vi "Calibrare.vi"() -> ()   [LabVIEW 2018]
panel:
  out "Timer":dbl
  out "Timer pornire":dbl
  out "Timer finalizare calibrare":dbl
  in  "Bluetooth":refnum<visa-resource-name>="COM3"
  in  "Perioada achizitie [s]":dbl=6.0 format="%#_13g"
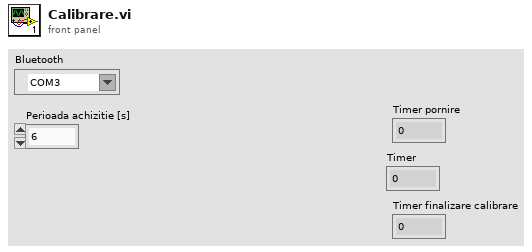
[diagram p1: front panel]
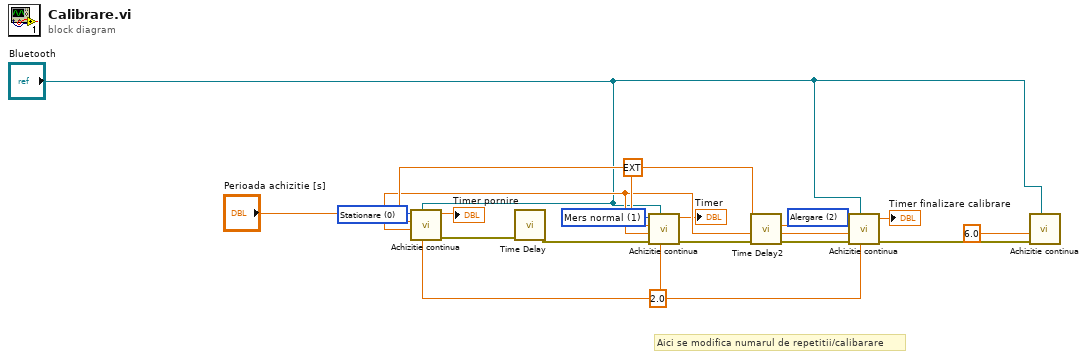
[diagram p0: block diagram]
diagram:
  w9 = 2.0 ("Numãrul de repetari")
  w11 = ext 99.0 ("Numarul persoanei")
  w12 = u16 2 items=["Stationare", "Mers normal", "Alergare", "Cadere", "Mers labartat"] ("Alegere Modul")
  w13 = u16 1 items=["Stationare", "Mers normal", "Alergare", "Cadere", "Mers labartat"] ("Alegere Modul")
  w14 = u16 0 items=["Stationare", "Mers normal", "Alergare", "Cadere", "Mers labartat"] ("Alegere Modul")
  # "Aici se modifica numarul de repetitii/calibarare"
  n1 = call "Achizitie continua.vi"("Numãrul de repetari"=w9, "Bluetooth"="Bluetooth", "Perioada achizitie [s]"="Perioada achizitie [s]", "Numarul persoanei"=w11, "Alegere Modul"=w14) -> ("error out"=w16:errorcluster, "Timer"=→"Timer pornire":dbl)  [unwired: 4 in]
  n2 = call "Time Delay"("error in (no error)"=w16) -> ("error out"=w3:errorcluster)  [unwired: 10 in]
  n3 = call "Achizitie continua.vi"("Numãrul de repetari"=w9, "Bluetooth"="Bluetooth", "error in (no error)"=w3, "Perioada achizitie [s]"="Perioada achizitie [s]", "Numarul persoanei"=w11, "Alegere Modul"=w13) -> ("error out"=w15:errorcluster, "Timer"=→"Timer":dbl)  [unwired: 3 in]
  n4 = call "Time Delay2"("error in (no error)"=w15) -> ("error out"=w2:errorcluster)  [unwired: 10 in]
  n5 = call "Achizitie continua.vi"("Numãrul de repetari"=w9, "Bluetooth"="Bluetooth", "error in (no error)"=w2, "Perioada achizitie [s]"="Perioada achizitie [s]", "Numarul persoanei"=w11, "Alegere Modul"=w12) -> ("error out"=w8:errorcluster, "Timer"=→"Timer finalizare calibrare":dbl)  [unwired: 3 in]
  n6 = call "Achizitie continua.vi"("Bluetooth"="Bluetooth", "error in (no error)"=w8, "Perioada achizitie [s]"=6.0) -> ()  [unwired: 6 in, 2 out]
